vi "oa_Remove DC Gap Reference (1 Channel).vi"(0 "resampled signal":cluster{"r0":dbl, "dr":dbl, "Y":dbl[]}={"r0"=0.0, "dr"=1.0, "Y"=[]} {"r0" format="%.2p"; "dr" format="%.2p"; "Y" format="%.2f"}, 1 "reset?":bool=TRUE, 2 "DC ref changed?":bool=TRUE, 5 "DC gap reference [V]":dbl=inf, 11 "error in":errorcluster, 12 "averaging type":enum16{"Linear", "Exponential"}(ring), 13 "window":T1(ring)) -> (4 "DC value out":dbl[](array[numeric]), 8 "actual gap ref":dbl format="%.2f", 15 "error out":errorcluster)   [LabVIEW 2017, in "SoundVib_RefDataProcess.lvlib"]
uses:
  <vilib>/addons/Sound and Vibration/Order Analysis/Referece Data Processing/SoundVib_RefDataProcess.lvlib
  <vilib>/measure/madcrms.llb/Basic Averaged DC-RMS for 1 Chan.vi
  <vilib>/measure/NI_MAPro.lvlib
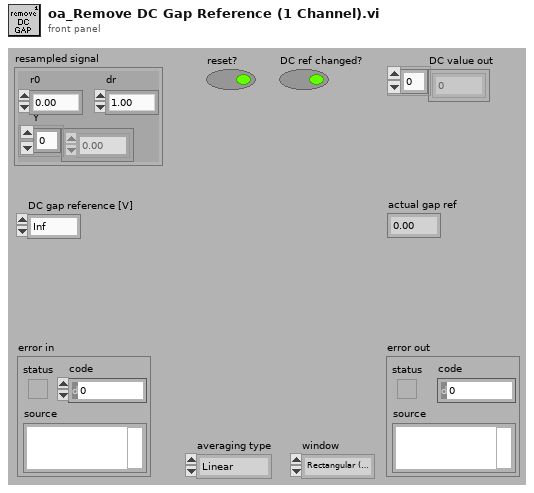
[diagram p1: front panel]
types:
  T1 = enum16{"Rectangular (none)", "Hanning", "Low side lobe"}
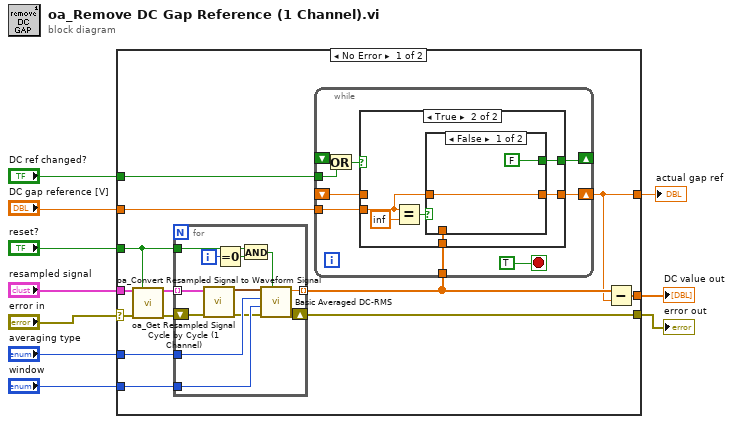
[diagram p0: block diagram]
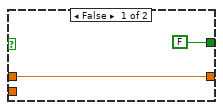
[diagram p2: hidden frame]
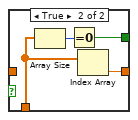
[diagram p3: hidden frame]
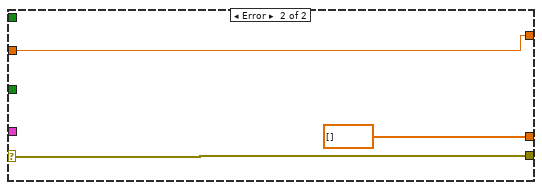
[diagram p4: hidden frame]
diagram:
  n1 = case shown="No Error" "error in" {
    selector: "error in" -> [w17 w61]
    tunnel: [w23 dbl[] []] -> w10
    tunnel: [w15 w61] -> w9
    tunnel: "window" -> [w22 _]
    tunnel: "averaging type" -> [w21 _]
    tunnel: "DC gap reference [V]" -> [w20 w59]
    tunnel: "reset?" -> [w13 _]
    tunnel: "DC ref changed?" -> [w19 _]
    tunnel: "resampled signal" -> [w18 _]
    tunnel: [w11 w59] -> w1
    frame No Error {
      n2 = call <vilib>:"oa_Get Resampled Signal Cycle by Cycle (1 Channel).vi"("resampled signal"=w18, "reset?"=w13, "error in"=w17) -> ("signal out"=w14:cluster{"r0":dbl, "dr":dbl, "Y":dbl[]}[], "error out"=w16:errorcluster)  [unwired: 11 in]
      n3 = for {
        tunnel: w13 -> [w54]
        tunnel: w21 -> [w58]
        tunnel: w22 -> [w57]
        tunnel: [w52] -> w12 mode=indexing
        shift-right: [w47] -> w15
        shift-left: w16 -> [w51]
        tunnel: w14 -> [w49] mode=indexing
        i -> [w56]
        n4 = call <vilib>:"oa_Convert Resampled Signal to Waveform Signal.vi"("resampled signal"=w49, "error in"=w51) -> ("signal in"=w48:waveform(dbl), "error out"=w50:errorcluster)  [unwired: 12 in]
        n5 = Equal To 0?(x=w56) -> (x = 0?=w55:bool)
        n6 = And(x=w54, y=w55) -> (x .and. y?=w53:bool)
        n7 = call-poly <vilib>:"Basic Averaged DC-RMS.vi"("reset"=w53, "error in (no error)"=w50, "window"=w57, "averaging type"=w58, "signal in"=w48) -> ("error out"=w47:errorcluster, "DC value"=w52:dbl)  [unwired: 3 in, 2 out]
      }
      n8 = while {
        tunnel: w20 -> [w32]
        tunnel: w19 -> [w26]
        shift-right: [w30] -> w11
        shift-left: _ -> [w29]
        tunnel: w12 -> [w28]
        shift-right: [w25] -> _
        shift-left: _ -> [w27]
        stop <- TRUE stop-if-true
        n9 = Or(x=w27, y=w26) -> (x .or. y?=w24:bool)
        n10 = case shown="True" w24 {
          tunnel: w32 -> [_ w38]
          tunnel: [w34 w37] -> w30
          tunnel: w29 -> [w34 _]
          tunnel: w28 -> [_ w36]
          tunnel: [FALSE w35] -> w25
          frame False {
          }
          frame True {
            n11 = Equal?(x=w38, y=inf) -> (x = y?=w39:bool)
            n12 = case shown="False" w39 {
              tunnel: [w42 w46] -> w37
              tunnel: w38 -> [w42 _]
              tunnel: w36 -> [_ w45]
              tunnel: [FALSE w43] -> w35
              frame False {
              }
              frame True {
                n13 = Array Size(array=w45) -> (size(s)=w44:i32)
                n14 = Equal To 0?(x=w44) -> (x = 0?=w43:bool)
                n15 = Index Array(array=w45) -> (element=w46:dbl)  [unwired: 1 in]
              }
            }
          }
        }
      }
      n16 = Subtract(x=w12, y=w11) -> (x-y=w23:dbl[])
    }
    frame Error {
    }
  }
  "DC value out" <- w10
  "error out" <- w9
  "actual gap ref" <- w1
